vi "insertString.vi"(1 "input":string, 2 "index":i32, 3 "array":string[](array[string])) -> (0 "output array":string[](array[string]))   [LabVIEW 2013]
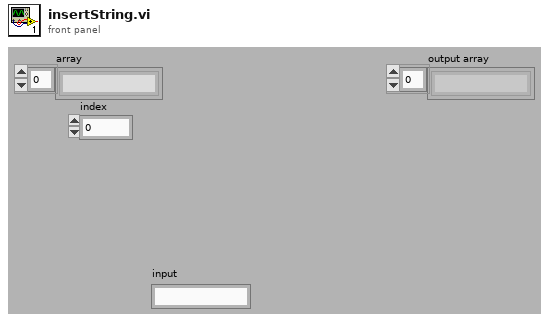
[diagram p1: front panel]
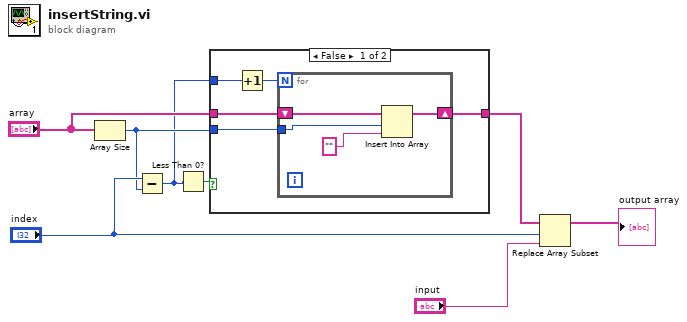
[diagram p0: block diagram]
diagram:
  n1 = Array Size(array="array") -> (size(s)=w3:i32)
  n2 = Subtract(x="index", y=w3) -> (x-y=w1:i32)
  n3 = Less Than 0?(x=w1) -> (x < 0?=w2:bool)
  n4 = case shown="False" w2 {
    tunnel: "array" -> [w12 w18]
    tunnel: [w13 w18] -> w5
    tunnel: w1 -> [w10 _]
    tunnel: w3 -> [w9 _]
    frame False {
      n5 = Increment(x=w10) -> (x+1=w11:i32)
      n6 = for {
        N: w11 -> [_]
        shift-right: [w16] -> w13
        shift-left: w12 -> [w17]
        tunnel: w9 -> [w15]
        n7 = Insert Into Array(array=w17, index=w15, new element="") -> (w16:string[])
      }
    }
    frame True {
    }
  }
  n8 = Replace Array Subset(array=w5, new element="input", index="index") -> (→"output array":string[])
